vi "Save Settings to XML.vi"(8 "error in (no error)":errorcluster, 10 "SaveDefault=false":bool, 11 "Settings":T1 {"Hardware Configuration"."Lasers Configuration"."SettingValues"."785 Power" format="%.1f"; "Hardware Configuration"."Lasers Configuration"."SettingValues"."647 Power" format="%.1f"; "Hardware Configuration"."Lasers Configuration"."SettingValues"."561 Power" format="%.1f"; "Hardware Configuration"."Lasers Configuration"."SettingValues"."532 Power" format="%.1f"; "Hardware Configuration"."Lasers Configuration"."SettingValues"."488 Power" format="%.1f"; "Hardware Configuration"."Lasers Configuration"."SettingValues"."405 Power" format="%.1f"}) -> (0 "error out":errorcluster, 3 "Settings Out":T1 {"Hardware Configuration"."Lasers Configuration"."SettingValues"."785 Power" format="%.1f"; "Hardware Configuration"."Lasers Configuration"."SettingValues"."647 Power" format="%.1f"; "Hardware Configuration"."Lasers Configuration"."SettingValues"."561 Power" format="%.1f"; "Hardware Configuration"."Lasers Configuration"."SettingValues"."532 Power" format="%.1f"; "Hardware Configuration"."Lasers Configuration"."SettingValues"."488 Power" format="%.1f"; "Hardware Configuration"."Lasers Configuration"."SettingValues"."405 Power" format="%.1f"})   [LabVIEW 2019, in "Settings.lvlib"]
doc: "Saves the \"User Specified\" configuration data to an XML file. This is used to remember the users settings between executions."
uses:
  Settings.lvlib
  Settings.ctl
  HardwareAdapter/Support/Hardware Configuration.ctl
  HardwareAdapter/Support/Camera Configuration.ctl
  D:/SDK/PMQI-LabViewSamples/Examples/Dependencies/PVCamNET.dll
  <vilib>/userdefined/High Color/IMAQdx.ctl
  E:/DevHardSoftware/MMicroscopy/HardwareAdapter/Lasers/Dependencies/Oxxius_Boxx.dll
  HardwareAdapter/Lasers/Dependencies/Oxxius_Boxx.dll
  Logging/Logging Configuration.ctl
  controls/UI Configuration.ctl
  <vilib>/Utility/xml.llb/Write to XML File(string).vi
  Logging/Logging.lvlib
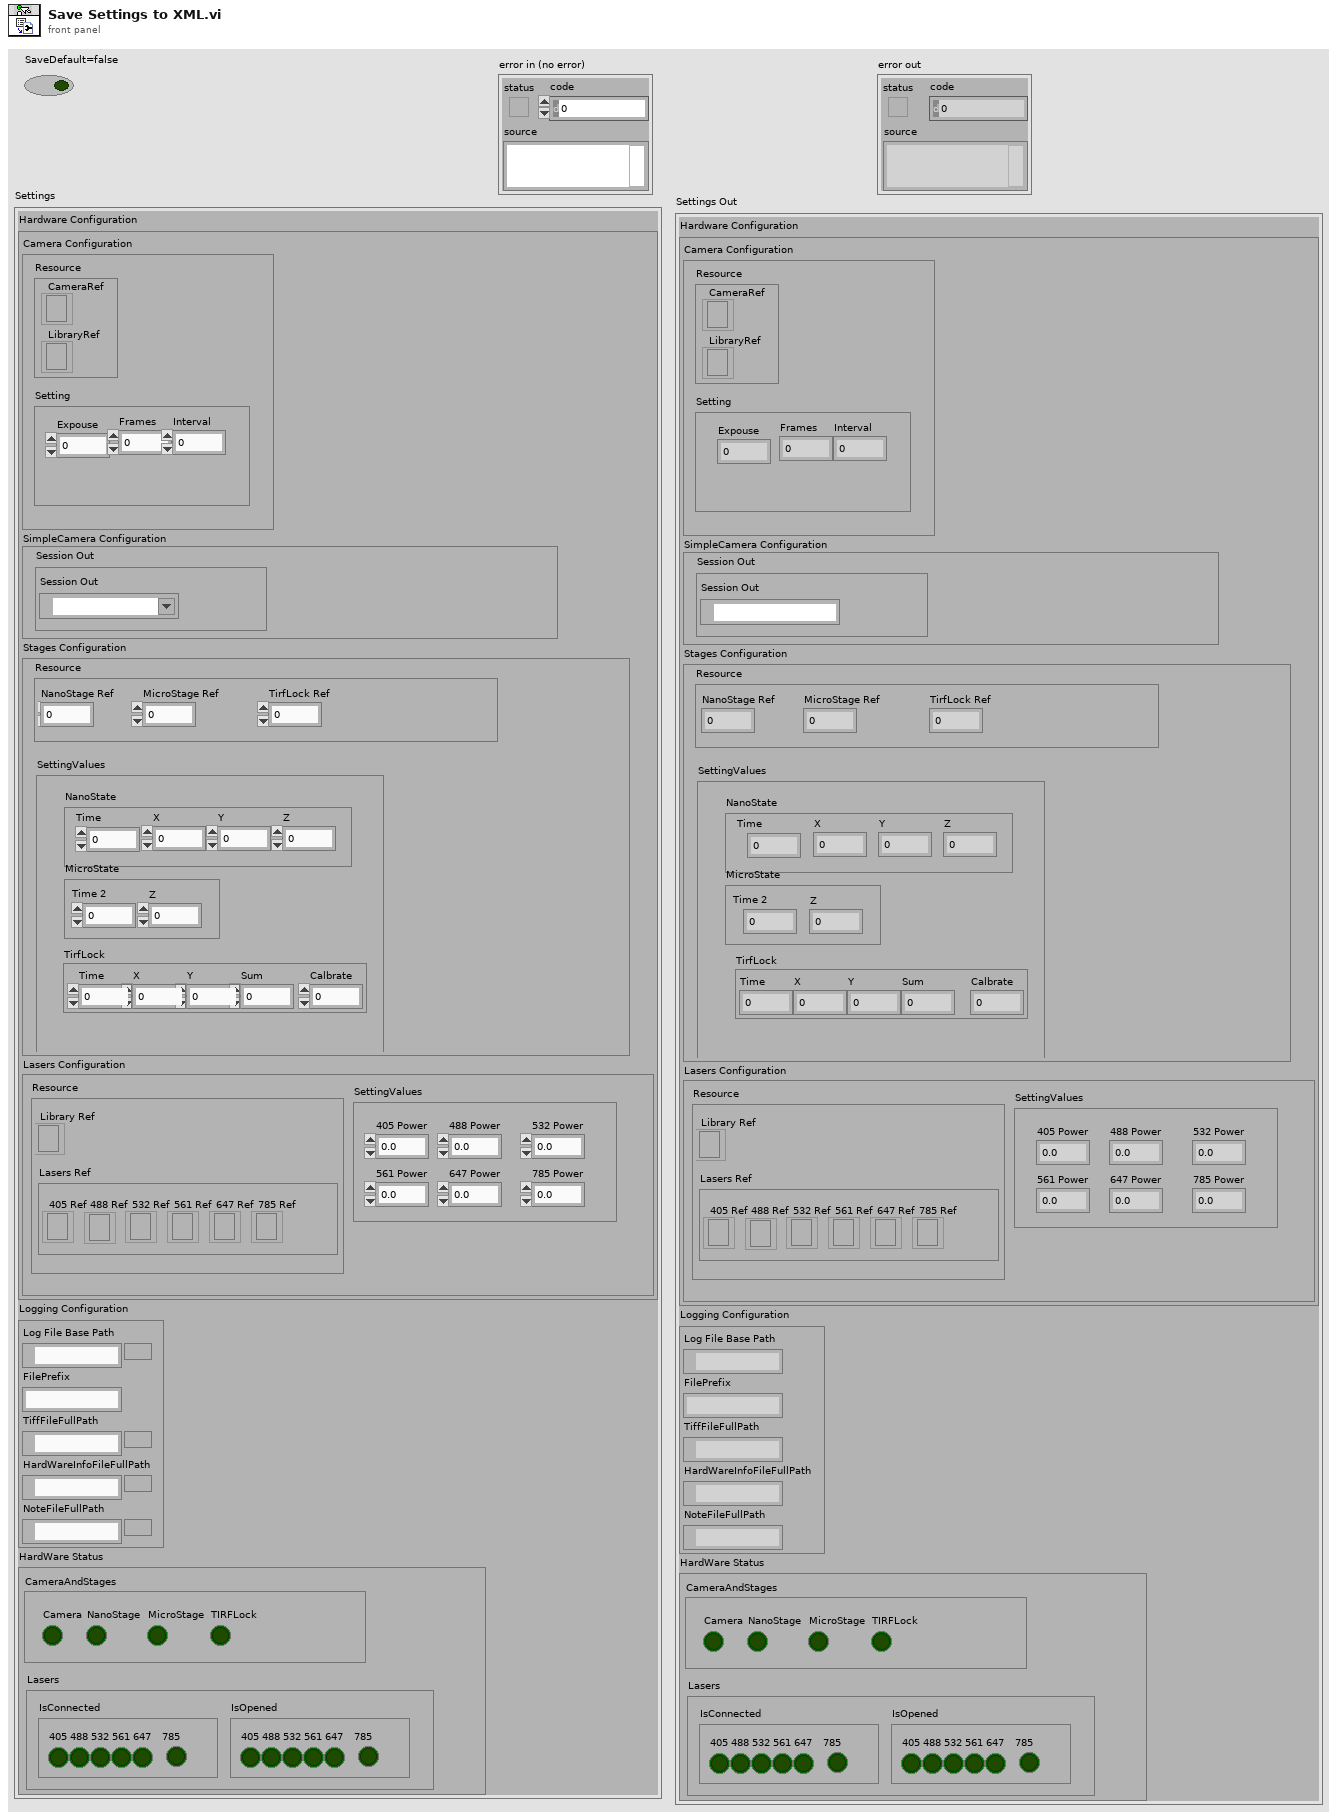
[diagram p1: front panel]
types:
  T1 = typedef "Settings.lvlib/Settings.ctl" = cluster{"Hardware Configuration":T2, "Logging Configuration":T5, "HardWare Status":cluster{"CameraAndStages":T6, "Lasers":cluster{"IsConnected":cluster{"405":bool, "488":bool, "532":bool, "561":bool, "647":bool, "785":bool}, "IsOpened":cluster{"405":bool, "488":bool, "532":bool, "561":bool, "647":bool, "785":bool}}}}
  T2 = typedef "Hardware Configuration.ctl" = cluster{"Camera Configuration":T3, "SimpleCamera Configuration":cluster{"Resource":cluster{"Session Out":T4}}, "Stages Configuration":cluster{"Resource":cluster{"NanoStage Ref":i32, "MicroStage Ref":i32, "TirfLock Ref":i32}, "SettingValues":cluster{"NanoState":cluster{"Time":dbl, "X":dbl, "Y":dbl, "Z":dbl}, "MicroState":cluster{"Time 2":dbl, "Z":dbl}, "TirfLock":cluster{"Time":dbl, "X":dbl, "Y":dbl, "Sum":dbl, "Calbrate":dbl}}}, "Lasers Configuration":cluster{"SettingValues":cluster{"405 Power":sgl, "488 Power":sgl, "532 Power":sgl, "561 Power":sgl, "647 Power":sgl, "785 Power":sgl}, "Resource":cluster{"Library Ref":refnum<k24>, "Lasers Ref":cluster{"405 Ref":refnum<k24>, "488 Ref":refnum<k24>, "532 Ref":refnum<k24>, "561 Ref":refnum<k24>, "647 Ref":refnum<k24>, "785 Ref":refnum<k24>}}}}
  T3 = typedef "Camera Configuration.ctl" = cluster{"Resource":cluster{"CameraRef":refnum<k24>, "LibraryRef":refnum<k24>}, "Setting":cluster{"Expouse":dbl, "Frames":dbl, "Interval":dbl}}
  T4 = typedef "IMAQdx.ctl" = refnum<k21>
  T5 = typedef "Logging.lvlib/Logging Configuration.ctl" = cluster{"Log File Base Path":path, "FilePrefix":string, "TiffFileFullPath":path, "HardWareInfoFileFullPath":path, "NoteFileFullPath":path}
  T6 = typedef "UI Configuration.ctl" = cluster{"Camera":bool, "NanoStage":bool, "MicroStage":bool, "TIRFLock":bool}
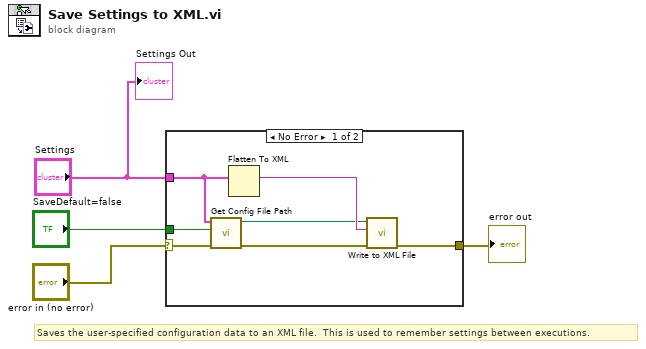
[diagram p0: block diagram]
diagram:
  # "Saves the user-specified configuration data to an XML file.  This is used to remember settings between executions."
  n1 = case shown="No Error" "error in (no error)" {
    selector: "error in (no error)" -> [w8 w12]
    tunnel: [w10 w12] -> w3
    tunnel: "Settings" -> [w6 _]
    tunnel: "SaveDefault=false" -> [w5 _]
    frame No Error {
      n2 = call "Get Config File Path.vi"("error in (no error)"=w8, "SaveDefault=false"=w5, "Settings"=w6) -> ("error out"=w7:errorcluster, "XML File Path"=w9:path)  [unwired: 7 in]
      n3 = Flatten To XML(anything=w6) -> (xml string=w11:string)
      n4 = call-poly <vilib>:"Write to XML File.vi"("error in (no error)"=w7, "XML Input"=w11, "XML File Path"=w9) -> ("error out"=w10:errorcluster)  [unwired: 6 in, 2 out]
    }
    frame Error {
    }
  }
  "error out" <- w3
  "Settings Out" <- "Settings"
